vi "run.vi"(8 "error in (no error)":errorcluster, 11 "GenericDataCollection in":refnum<class "GenericDataCollection.lvclass">) -> (0 "error out":errorcluster, 3 "GenericDataCollection out":refnum<class "GenericDataCollection.lvclass">)   [LabVIEW 2010, in "GenericDataCollection.lvclass"]
uses:
  GenericDataCollection.lvclass
  common/classes/GenericToplevelComponent/GenericToplevelComponent/common_trigger_enum.ctl
  common/classes/GenericToplevelComponent/GenericToplevelComponent/GenericToplevelComponent.lvclass
panel:
  # "Functionality not available..."
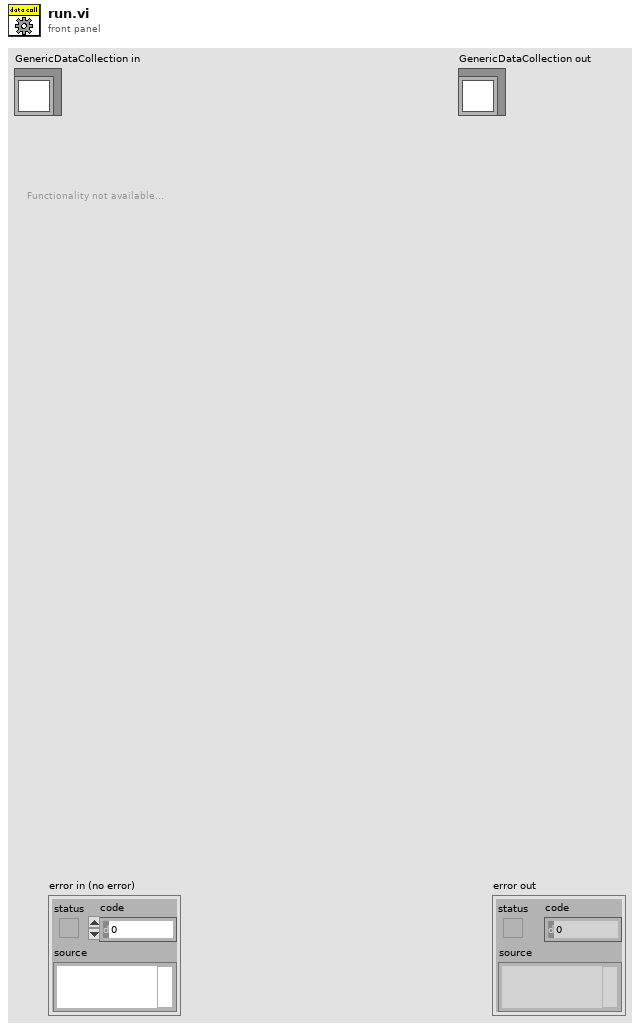
[diagram p1: front panel]
types:
  T1 = typedef "GenericToplevelComponent.lvclass/common_trigger_enum.ctl" = enum16{"NULL", "initialise", "terminate", "fetch command", "fetch data", "attach observer", "register as observer", "detach observer", "acknowledge", "start", "stop", "sweep started", "sweep finished", "experiment started", "experiment stopped"}
  T2 = typedef "main_trigger_enum.ctl" = enum16{"NULL", "initialise", "terminate", "start", "stop", "change objective", "change experimentController", "change imagingMode", "save notebook", "started saving", "finished saving", "expCtr ready", "expCtr missing", "imgMd ready", "imgMd missing", "scanHd ready", "scanHd missing", "DAQ ready", "DAQ missing", "imgAsm ready", "imgAsm missing", "dataColl ready", "dataColl missing", "display ready", "display missing", "analysr ready", "analysr missing", "instrmnt ready", "instrmnt missing", "stimltr ready", "stimltr missing", "stage ready", "stage missing"}
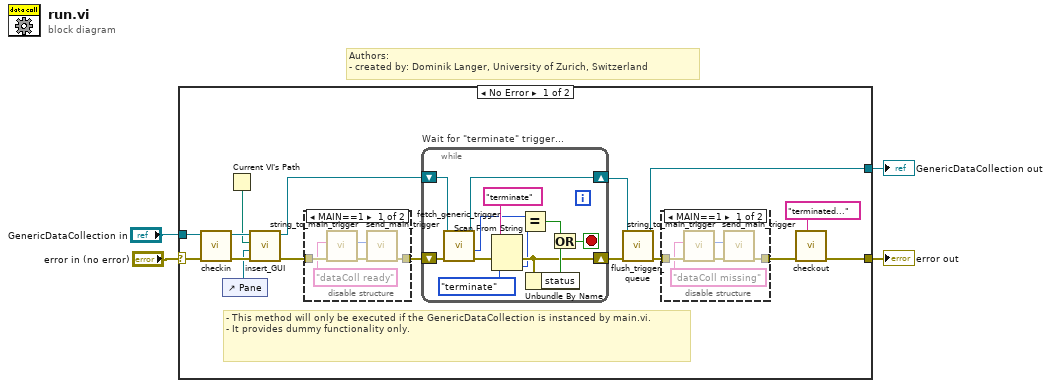
[diagram p0: block diagram]
diagram:
  # "Authors: \n- created by: Dominik Langer, University of Zurich, Switzerland"
  n1 = case shown="No Error" "error in (no error)" {
    selector: "error in (no error)" -> [w20 w46]
    tunnel: [w19 w46] -> w3
    tunnel: [w12 w45] -> w1
    tunnel: "GenericDataCollection in" -> [w18 w45]
    frame No Error {
      # "- This method will only be executed if the GenericDataCollection is instanced by main.vi.\n- It provides dummy functionality only."
      n2 = call-dynamic "checkin.vi"("error in (no error)"=w20, "GenericDataCollection in"=w18) -> ("error out"=w16:errorcluster, "GenericDataCollection out"=w17:refnum<class "GenericDataCollection.lvclass">)  [unwired: 8 in]
      n3 = control-ref of="Pane"() -> (w14:refnum<vi>)
      n4 = Current VI's Path() -> (path=w15:path)
      n5 = call-dynamic "insert_GUI.vi"("error in (no error)"=w16, "Pane"=w14, "VI path"=w15, "GenericComponent in"=w17) -> ("error out"=w8:errorcluster, "GenericComponent out"=w13:refnum<class "GenericDataCollection.lvclass">)  [unwired: 6 in]
      n6 = disable-structure shown="MAIN==1" {
        disable-tunnel: [w31 w32] -> w5
        disable-tunnel: w8 -> [w30 w32]
        frame condition #0 {
          n7 = call "string_to_main_trigger.vi"("error in (no error)"=w30, "trigger string"="dataColl ready") -> ("error out"=w29:errorcluster, "main trigger"=w28:T2)  [unwired: 8 in]
          n8 = call "send_main_trigger.vi"("error in (no error)"=w29, "trigger"=w28) -> ("error out"=w31:errorcluster)  [unwired: 9 in]
        }
        frame condition #1 (active) {
        }
      }
      n9 = while "Wait for \"terminate\" trigger..." {
        shift-right: [w36] -> w11
        shift-left: w5 -> [w44]
        shift-right: [w42] -> w10
        shift-left: w13 -> [w43]
        stop <- w40 stop-if-true
        n10 = call-dynamic "fetch_generic_trigger.vi"("error in (no error)"=w44, "GenericToplevelComponent in"=w43) -> ("error out"=w37:errorcluster, "common trigger"=w38:T1, "GenericToplevelComponent out"=w42:refnum<class "GenericDataCollection.lvclass">)  [unwired: 3 in, 4 out]
        n11 = Scan From String(input string="terminate", error in=w37, default 1=common_trigger_enum."terminate" ("x")) -> (error out=w36:errorcluster, output 1=w34:T1)  [unwired: 2 in, 2 out]
        n12 = Equal?(x=w38, y=w34) -> (x = y?=w33:bool)
        n13 = Unbundle By Name(w36) -> ("status"=w41:bool)
        n14 = Or(x=w33, y=w41) -> (x .or. y?=w40:bool)
      }
      n15 = call-dynamic "flush_trigger_queue.vi"("error in (no error)"=w11, "GenericToplevelComponent in"=w10) -> ("error out"=w6:errorcluster, "GenericToplevelComponent out"=w12:refnum<class "GenericDataCollection.lvclass">)  [unwired: 8 in]
      n16 = disable-structure shown="MAIN==1" {
        disable-tunnel: [w25 w26] -> w7
        disable-tunnel: w6 -> [w24 w26]
        frame condition #0 {
          n17 = call "string_to_main_trigger.vi"("error in (no error)"=w24, "trigger string"="dataColl missing") -> ("error out"=w23:errorcluster, "main trigger"=w22:T2)  [unwired: 8 in]
          n18 = call "send_main_trigger.vi"("error in (no error)"=w23, "trigger"=w22) -> ("error out"=w25:errorcluster)  [unwired: 9 in]
        }
        frame condition #1 (active) {
        }
      }
      n19 = call "checkout.vi"("locked by?"="terminated...", "error in (no error)"=w7) -> ("error out"=w19:errorcluster)  [unwired: 8 in, 1 out]
    }
    frame Error {
    }
  }
  "error out" <- w3
  "GenericDataCollection out" <- w1
